vi "_DoMultipleLCInjections.vi"(2 "# of Injections":u16, 3 "FirstCall (F)":bool) -> ()   [LabVIEW 2015]
uses:
  Type/_Log Command.ctl
  Type/_LC Command.ctl
  Server/_Server Global.vi
  _Global LC Driver.vi
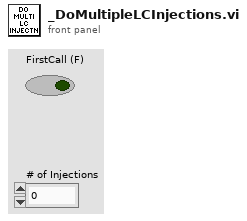
[diagram p1: front panel]
types:
  T1 = typedef "_Log Command.ctl" = enum16{"No Command", "Open", "Read", "Write", "Close", "Check Size"}
  T2 = typedef "_LC Command.ctl" = enum16{"No Command", "Initialize", "Get Configuration", "Get Status", "Get LC Method Contents", "Oven OnOff", "Pump OnOFF", "Rinse Autosampler", "Run Sample", "Set EnvParameters", "Set Method", "Start Equilibration", "Stop Run", "Get LastError", "Clear Error", "Close"}
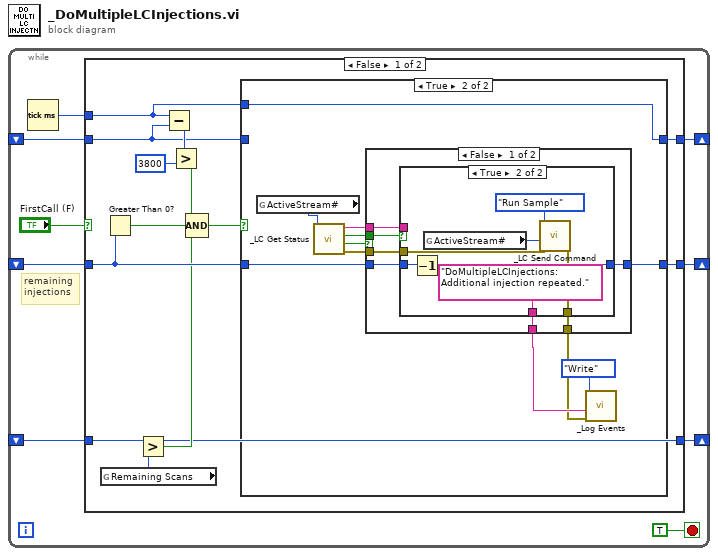
[diagram p0: block diagram]
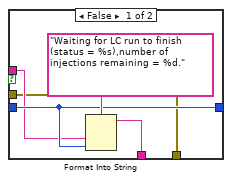
[diagram p3: hidden frame]
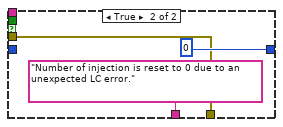
[diagram p4: hidden frame]
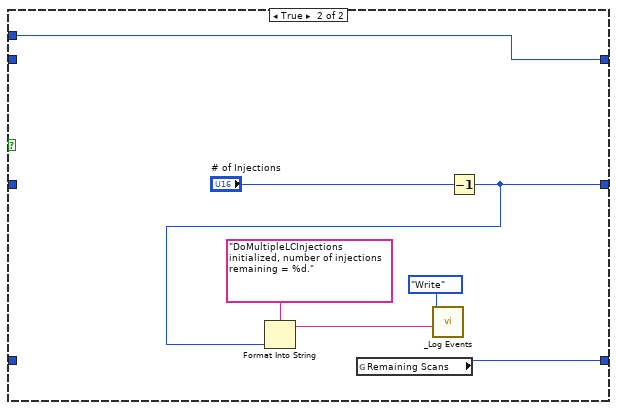
[diagram p5: hidden frame]
diagram:
  n1 = while {
    shift-right: [w7] -> _
    shift-left: _ -> [w6]
    shift-right: [w5] -> _
    shift-left: _ -> [w3]
    shift-right: [w2] -> _
    shift-left: _ -> [w1]
    stop <- TRUE stop-if-true
    # "remaining\ninjections"
    n2 = Tick Count (ms)() -> (millisecond timer value=w4:u32)
    n3 = case shown="False" "FirstCall (F)" {
      tunnel: [w21 w60] -> w7
      tunnel: w6 -> [w22 _]
      tunnel: [w14 w63] -> w5
      tunnel: w4 -> [w13 w63]
      tunnel: w3 -> [w15 _]
      tunnel: [w10 w58] -> w2
      tunnel: w1 -> [w10 _]
      frame False {
        n4 = global read "_Server Global.vi" "Remaining Scans"() -> (w12:i32)
        n5 = Greater Than 0?(x=w22) -> (x > 0?=w18:bool)
        n6 = Greater?(x=w10, y=w12) -> (0:w11:bool)
        n7 = Subtract(x=w13, y=w15) -> (x-y=w20:u32)
        n8 = Greater?(x=w20, y=u32 3800) -> (0:w17:bool)
        n9 = Compound Arithmetic op=AND(w17, w18, w11) -> (w16:bool)
        n10 = case shown="True" w16 {
          tunnel: w22 -> [w24 w35]
          tunnel: [w24 w34] -> w21
          tunnel: [w23 w33] -> w14
          tunnel: w15 -> [w23 _]
          tunnel: w13 -> [_ w33]
          frame False {
          }
          frame True {
            n11 = global read "_Global LC Driver.vi" "ActiveStream#"() -> (w30:u8)
            n12 = call "_LC Get Status.vi"("Stream#"=w30) -> ("error out"=w26:errorcluster, "Error"=w29:bool, "Ready"=w28:bool, "LC Status"=w27:string)  [unwired: 3 in, 1 out]
            n13 = case shown="False" w29 {
              tunnel: [w40 u16 0] -> w34
              tunnel: w28 -> [w42 _]
              tunnel: w35 -> [w41 _]
              tunnel: [w39 "Number of injection is reset to 0 due to an unexpected LC error."] -> w31
              tunnel: w27 -> [w38 _]
              tunnel: w26 -> [w37 w55]
              tunnel: [w36 w55] -> w25
              frame False {
                n14 = case shown="True" w42 {
                  tunnel: w41 -> [w45 w54]
                  tunnel: [w45 w53] -> w40
                  tunnel: [w47 "DoMultipleLCInjections: Additional injection repeated."] -> w39
                  tunnel: w38 -> [w44 _]
                  tunnel: w37 -> [w43 w49]
                  tunnel: [w43 w48] -> w36
                  frame False {
                    n15 = Format Into String(format string="Waiting for LC run to finish (status = %s),number of injections remaining = %d.", w44, w45) -> (resulting string=w47:string)  [unwired: 2 in, 1 out]
                  }
                  frame True {
                    n16 = Decrement(x=w54) -> (x-1=w53:u16)
                    n17 = global read "_Global LC Driver.vi" "ActiveStream#"() -> (w51:u8)
                    n18 = call "_LC Send Command.vi"("error in"=w49, "Stream#"=w51, "Command"=_LC_Command."Run Sample") -> ("error out"=w48:errorcluster)  [unwired: 7 in, 1 out]
                  }
                }
              }
              frame True {
              }
            }
            n19 = call "_Log Events.vi"("error in (no error)"=w25, "Event"=w31, "Log Command"=_Log_Command."Write") -> ()  [unwired: 4 in, 2 out]
          }
        }
      }
      frame True {
        n20 = global read "_Server Global.vi" "Remaining Scans"() -> (w58:i32)
        n21 = Decrement(x="# of Injections") -> (x-1=w60:u16)
        n22 = Format Into String(format string="DoMultipleLCInjections initialized, number of injections remaining = %d.", w60) -> (resulting string=w59:string)  [unwired: 2 in, 1 out]
        n23 = call "_Log Events.vi"("Event"=w59, "Log Command"=_Log_Command."Write") -> ()  [unwired: 5 in, 2 out]
      }
    }
  }
